vi "Simulation Lab -data cluster - B220061.vi"() -> ()   [LabVIEW 2020]
panel:
  out "Gender 3":bool
  out "Name 3":string
  out "Roll No. 3":dbl
  out "Cluster":T1
  in  "Gender":bool
  in  "Name":string
  in  "Roll No.":dbl
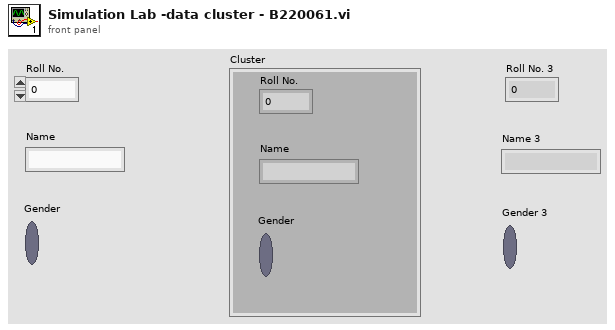
[diagram p1: front panel]
types:
  T1 = cluster{"Roll No.":dbl, "Name":string, "Gender":bool}
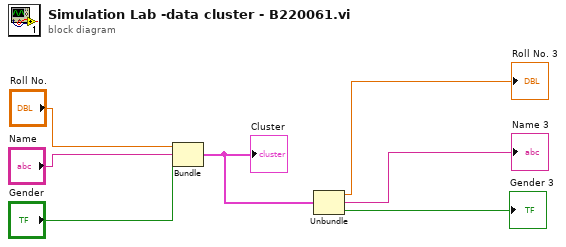
[diagram p0: block diagram]
diagram:
  n1 = Bundle "Bundle"("Roll No."="Roll No.", "Name"="Name", "Gender"="Gender") -> (w4:T1)  [unwired: 1 in]
  "Cluster" <- w4
  n2 = Unbundle "Unbundle"(w4) -> ("Roll No."=→"Roll No. 3":dbl, "Name"=→"Name 3":string, "Gender"=→"Gender 3":bool)
